vi "ECOG-Start.vi"(0 "params":T1, 11 "error in (no error)":errorcluster) -> (4 "task out":refnum<k21>, 8 "nread":i32, 15 "error out":errorcluster)   [LabVIEW 2020]
uses:
  Typedefs/ECOG-Parameters.ctl
  <vilib>/DAQmx/create/channels.llb/DAQmx Create Channel (AI-Voltage-Basic).vi
  <vilib>/DAQmx/configure/timing.llb/DAQmx Timing (Sample Clock).vi
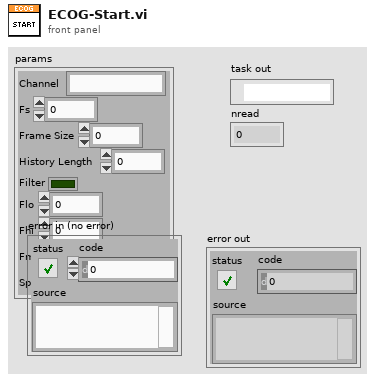
[diagram p1: front panel]
types:
  T1 = typedef "ECOG-Parameters.ctl" = cluster{"Channel":string, "Fs":dbl, "Frame Size":dbl, "History Length":dbl, "Filter":bool, "Flo":dbl, "Fhi":dbl, "Fmax":dbl, "Splitter Position":i32}
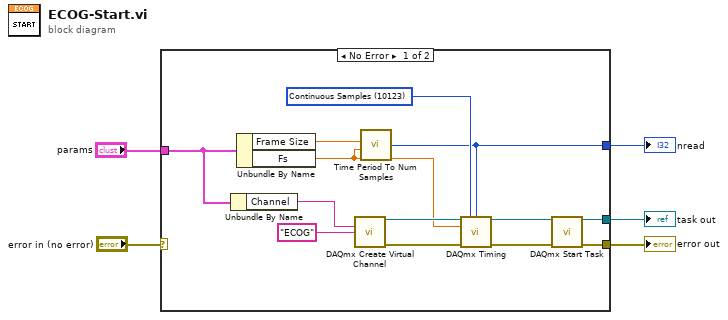
[diagram p0: block diagram]
diagram:
  n1 = case shown="No Error" "error in (no error)" {
    selector: "error in (no error)" -> [_ w19]
    tunnel: "params" -> [w14 _]
    tunnel: [w10 _] -> w4
    tunnel: [w7 w19] -> w3
    tunnel: [w6 _] -> w2
    frame No Error {
      w13 = 10123 items=["Finite Samples"=10178, "Continuous Samples"=10123, "Hardware Timed Single Point"=12522] ("sample mode")
      n2 = Unbundle By Name(w14) -> ("Channel"=w18:string)
      n3 = Unbundle By Name(w14) -> ("Frame Size"=w12:dbl, "Fs"=w11:dbl)
      n4 = call-poly <vilib>:"DAQmx Create Virtual Channel.vi"("physical channels"=w18, "name to assign"="ECOG") -> ("task out"=w16:refnum<k21>, "error out"=w15:errorcluster)  [unwired: 12 in]
      n5 = call "Time Period To Num Samples.vi"("Duration (ms)"=w12, "Sampling rate (Hz)"=w11) -> ("Samples"=w10:i32)  [unwired: 5 in]
      n6 = call-poly <vilib>:"DAQmx Timing.vi"("task/channels in"=w16, "sample mode"=w13, "samples per channel"=w10, "rate"=w11, "error in"=w15) -> ("task out"=w9:refnum<k21>, "error out"=w8:errorcluster)  [unwired: 9 in]
      n7 = call <vilib>:"DAQmx Start Task.vi"("task/channels in"=w9, "error in"=w8) -> ("task out"=w6:refnum<k21>, "error out"=w7:errorcluster)  [unwired: 12 in]
    }
    frame Error {
    }
  }
  "error out" <- w3
  "task out" <- w2
  "nread" <- w4
